vi "Eval_MultiVar_MultiRes.vi"(8 "error in (no error)":errorcluster, 9 "varValues":dbl[](array[numeric]) format="%#_13g", 10 "varNames":string[](array[string]), 11 "mupExpr in":refnum<data-value>) -> (0 "error out":errorcluster, 2 "Results":dbl[](array[numeric]) format="%#_13g", 3 "mupExpr out":refnum<data-value>)   [LabVIEW 2015, in "mupExpr.lvclass"]
doc: "Update the value of multiple variables then evaluate all expression. Returns one result per expression.\n\nIf any variable is not found, a warning is generated.\n\nIf the variables are defined for bulk mode evaluation, only the first set (index 0) will be updated and evaluated."
uses:
  mupExpr.lvclass
  mupExpr.lvclass/mupExpr.ctl
  mupLib/mupSetVarValue.vi
  mupLib/mupCheckError.vi
  mupLib/mupLibPath.vi
  <vilib>/Utility/error.llb/Error Cluster From Error Code.vi
  mupLib/mupLib.lvlib
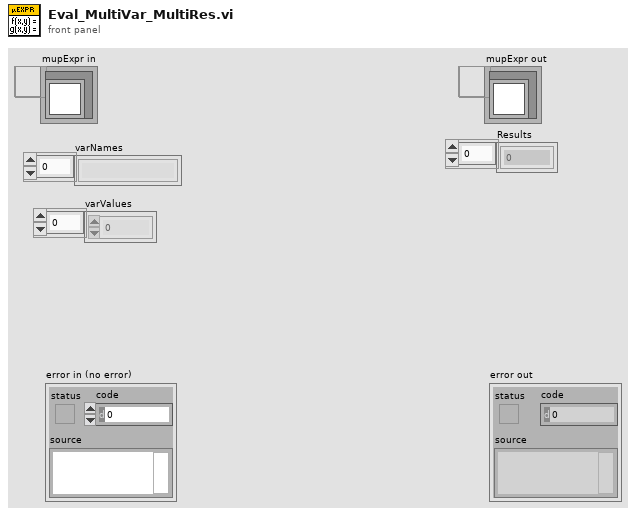
[diagram p1: front panel]
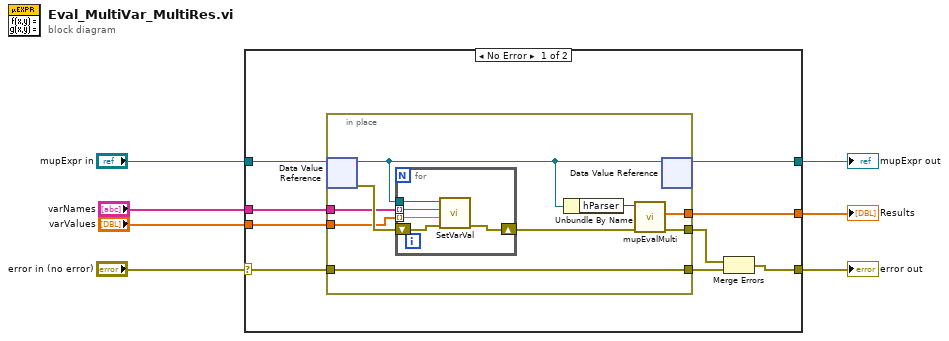
[diagram p0: block diagram]
diagram:
  n1 = case shown="No Error" "error in (no error)" {
    selector: "error in (no error)" -> [w8 w32]
    tunnel: "varValues" -> [w16 _]
    tunnel: "varNames" -> [w15 _]
    tunnel: [w14 _] -> w5
    tunnel: "mupExpr in" -> [w13 w31]
    tunnel: [w10 w32] -> w3
    tunnel: [w9 w31] -> w2
    frame No Error {
      n2 = in-place {
        in-place-border: w8 -> [w23]
        in-place-border: [w25] -> w11
        in-place-border: [w17] -> w14
        in-place-border: [w23] -> w12
        in-place-border: w16 -> [w20]
        in-place-border: w15 -> [w19]
        n3 = in-place-dvr #1(w13) -> (w18:refnum<class "mupExpr.lvclass">, w22:errorcluster)
        n4 = for {
          tunnel: w19 -> [w30] mode=indexing
          tunnel: w20 -> [w29] mode=indexing
          shift-right: [w27] -> w21
          shift-left: w22 -> [w28]
          tunnel: w18 -> [w26]
          n5 = call "SetVarVal.vi"("error in (no error)"=w28, "varValue"=w29, "varName"=w30, "muExpr in"=w26) -> ("error out"=w27:errorcluster)  [unwired: 6 in, 1 out]
        }
        n6 = Unbundle By Name(w18) -> ("hParser"=w24:u64)
        n7 = call "mupEvalMulti.vi"("error in (no error)"=w21, "hParser in"=w24) -> ("error out"=w25:errorcluster, "results"=w17:dbl[])  [unwired: 6 in, 2 out]
        n8 = in-place-dvr #1(w18) -> (w9:refnum<data-value>)  [unwired: 1 out]
      }
      n9 = Merge Errors(w11, w12) -> (w10:errorcluster)
    }
    frame Error {
    }
  }
  "error out" <- w3
  "mupExpr out" <- w2
  "Results" <- w5
